vi "FABR-Initialize Frequency Axis.vi"(0 "XYGraph in":refnum<vi>, 5 "FreqAxisLabel":refnum<vi>, 7 "Array":dbl[](array[numeric]), 11 "error in (no error)":errorcluster) -> (15 "error out":errorcluster)   [LabVIEW 2020]
uses:
  epl-vi-lib/Utility VIs/Math VIs/LinSpace (x0-dx-npts).vi
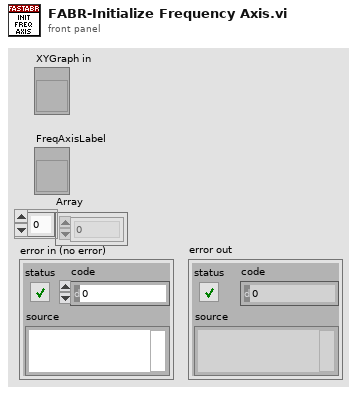
[diagram p1: front panel]
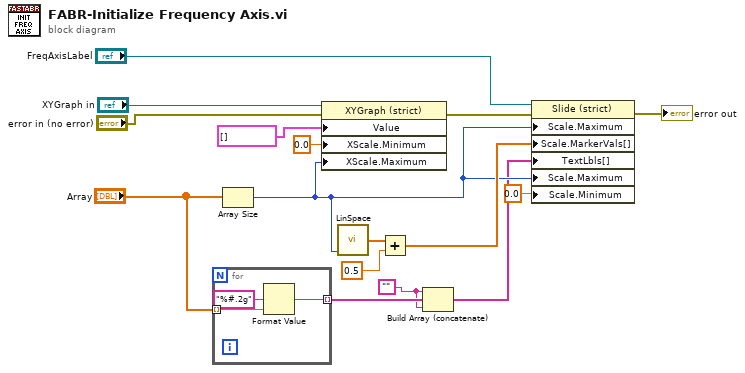
[diagram p0: block diagram]
diagram:
  w2 = ""
  n1 = for {
    tunnel: "Array" -> [w19] mode=indexing
    tunnel: [w17] -> w6 mode=indexing
    n2 = Format Value(format string="%#.2g", value (0)=w19) -> (output string=w17:string)  [unwired: 1 in]
  }
  n3 = Array Size(array="Array") -> (size(s)=w4:i32)
  n4 = property class="XYGraph (strict)"(reference="XYGraph in", error in="error in (no error)", "Value"=cluster{dbl[], dbl[]}[] [], "XScale.Minimum"=0.0 ("X Scale.Range:Maximum"), "XScale.Maximum"=w4) -> (error out=w12:errorcluster)  [unwired: 1 out]
  n5 = call-poly "LinSpace.vi"("npts"=w4) -> ("Array"=w11:dbl[])  [unwired: 3 in, 1 out]
  n6 = Add(x=w11, y=0.5) -> (x+y=w9:dbl[])
  n7 = Build Array (concatenate)(w2, w6, w2) -> (w3:string[])
  n8 = property class="Slide (strict)"(reference="FreqAxisLabel", error in=w12, "Scale.Maximum"=w4, "Scale.MarkerVals[]"=w9, "TextLbls[]"=w3, "Scale.Maximum"=w4, "Scale.Minimum"=0.0 ("Scale.Range:Minimum")) -> (error out=→"error out":errorcluster)  [unwired: 1 out]
